vi "Run I2C Script Directly.vi"(8 "error in":errorcluster, 9 "configuration scripts":path[](array[path]), 10 "serial channels":string[](array[string]), 11 "FPGA Ref In":refnum<k20>) -> (0 "error out":errorcluster, 3 "FPGA Ref Out":refnum<k20>)   [LabVIEW 2025, in "I2C Bus Monitor.lvclass"]
uses:
  I2C Bus Monitor.lvclass
  Error Global.vi
  I2C Bus Monitor.lvclass/I2C Bus Monitor.ctl
  <instrlib>/FlexRIO/API/Host/v1/NI FlexRIO API v1.lvlib
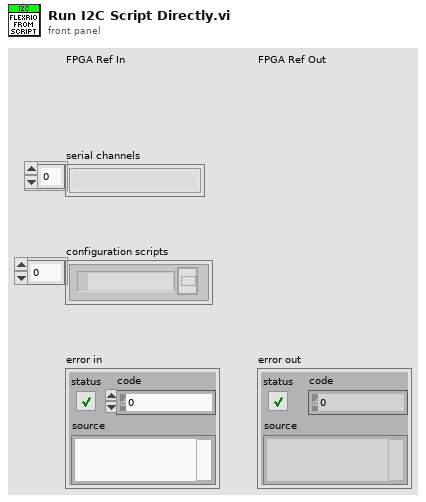
[diagram p1: front panel]
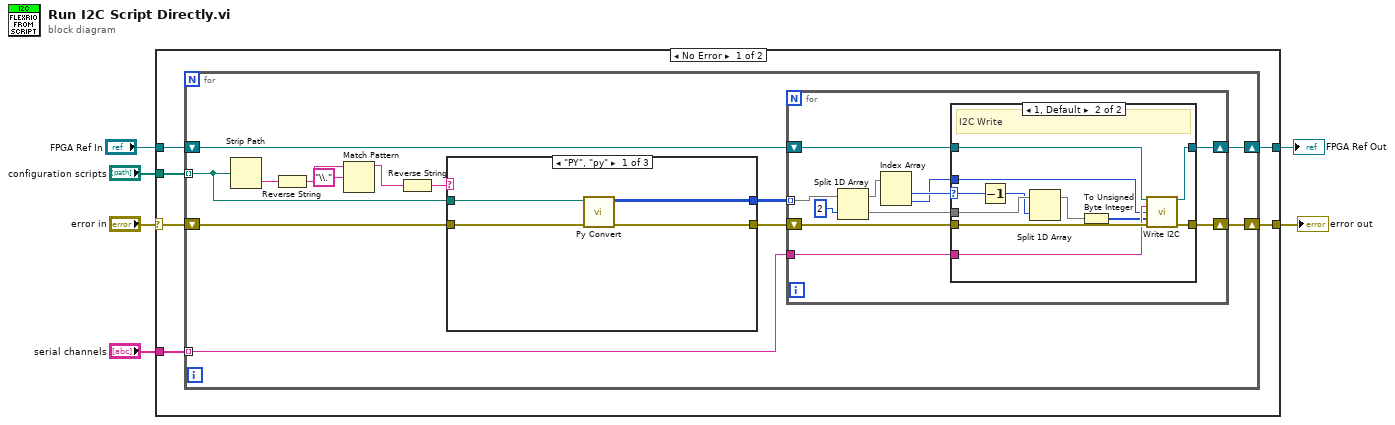
[diagram p0: block diagram]
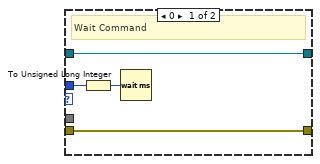
[diagram p2: hidden frame]
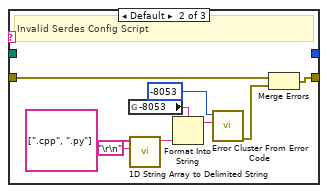
[diagram p3: hidden frame]
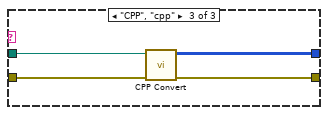
[diagram p4: hidden frame]
diagram:
  n1 = case shown="No Error" "error in" {
    selector: "error in" -> [w7 w70]
    tunnel: [w12 w70] -> w6
    tunnel: "serial channels" -> [w11 _]
    tunnel: "configuration scripts" -> [w10 _]
    tunnel: [w9 w69] -> w3
    tunnel: "FPGA Ref In" -> [w8 w69]
    frame No Error {
      n2 = for {
        tunnel: w11 -> [w13] mode=indexing
        tunnel: w10 -> [w22] mode=indexing
        shift-right: [w24] -> w12
        shift-left: w7 -> [w14]
        shift-right: [w16] -> w9
        shift-left: w8 -> [w15]
        n3 = Strip Path(path=w22) -> (name=w21:string)  [unwired: 1 out]
        n4 = Reverse String(1:w21) -> (0:w20:string)
        n5 = Match Pattern(string=w20, regular expression="\\.") -> (before substring=w18:string)  [unwired: 1 in, 3 out]
        n6 = Reverse String(1:w18) -> (0:w17:string)
        n7 = case shown="\"PY\", \"py\"" w17 {
          tunnel: [w52 _ w68] -> w25
          tunnel: w14 -> [w54 w64 w67]
          tunnel: w22 -> [w55 _ w66]
          tunnel: [w53 w63 w65] -> w23
          frame "PY", "py" {
            n8 = call "Py Convert.vi"("error in (no error)"=w54, "configuration scripts"=w55) -> ("error out"=w53:errorcluster, "I2C Commands"=w52:u16[][])  [unwired: 8 in]
          }
          frame Default {
            # "Invalid Serdes Config Script"
            n9 = global read "Error Global.vi" "-8053"() -> (w62:string)
            n10 = call <vilib>:"1D String Array to Delimited String.vi"("delimiter"="\r\n", "string array"=string[] [".cpp", ".py"]) -> ("delimited string"=w59:string)  [unwired: 9 in]
            n11 = Format Into String(format string=w62, w59) -> (resulting string=w61:string)  [unwired: 2 in, 1 out]
            n12 = call <vilib>:"Error Cluster From Error Code.vi"("error message (\"\")"=w61, "error code (0)"=-8053) -> ("error out"=w58:errorcluster)  [unwired: 7 in]
            n13 = Merge Errors(w64, w58) -> (w63:errorcluster)
          }
          frame "CPP", "cpp" {
            n14 = call "CPP Convert.vi"("error in (no error)"=w67, "configuration scripts"=w66) -> ("error out"=w65:errorcluster, "I2C Commands"=w68:u16[][])  [unwired: 8 in]
          }
        }
        n15 = for {
          tunnel: w25 -> [w36] mode=indexing
          shift-right: [w29] -> w24
          shift-left: w23 -> [w30]
          tunnel: w13 -> [w27]
          shift-right: [w26] -> w16
          shift-left: w15 -> [w28]
          n16 = Split 1D Array(array=w36, index=2) -> (first subarray=w34:u16[], second subarray=w32:u16[])
          n17 = Index Array(array=w34) -> (element #1=w33:u16, element #2=w31:u16)  [unwired: 2 in]
          n18 = case shown="1, Default" w33 {
            selector: w33 -> [_ w51]
            tunnel: w32 -> [_ w50]
            tunnel: w31 -> [w40 w44]
            tunnel: w30 -> [w39 w48]
            tunnel: [w39 w47] -> w29
            tunnel: w28 -> [w37 w46]
            tunnel: w27 -> [_ w45]
            tunnel: [w37 w41] -> w26
            frame 0 {
              # "Wait Command"
              n19 = To Unsigned Long Integer(number=w40) -> (unsigned 32bit integer=w38:u32)
              n20 = Wait (ms)(milliseconds to wait=w38) -> ()  [unwired: 1 out]
            }
            frame 1, Default {
              # "I2C Write"
              n21 = Decrement(x=w51) -> (x-1=w49:u16)
              n22 = Split 1D Array(array=w50, index=w49) -> (first subarray=w43:u16[])  [unwired: 1 out]
              n23 = To Unsigned Byte Integer(number=w43) -> (unsigned 8bit integer=w42:u8[])
              n24 = call <instrlib>:"Write I2C.vi"("fpga interface in"=w46, "bus instance name"=w45, "slave address"=w44, "data"=w42, "error in"=w48) -> ("fpga interface out"=w41:refnum<k20>, "error out"=w47:errorcluster)  [unwired: 8 in, 1 out]
            }
          }
        }
      }
    }
    frame Error {
    }
  }
  "error out" <- w6
  "FPGA Ref Out" <- w3
